vi "Export Custom Device Configuration.vi"(8 "error in (no error)":errorcluster, 11 "Node Ptr":u64 format="%.0x") -> (0 "error out":errorcluster)   [LabVIEW 2015, in "Import Export Sample Custom Device System Explorer.lvlib"]
uses:
  Import Export Sample Custom Device System Explorer.lvlib
  <vilib>/NI/NIVS System Definition Utilities/System Definition Utilities.lvlib
panel:
  in  "Tag":string
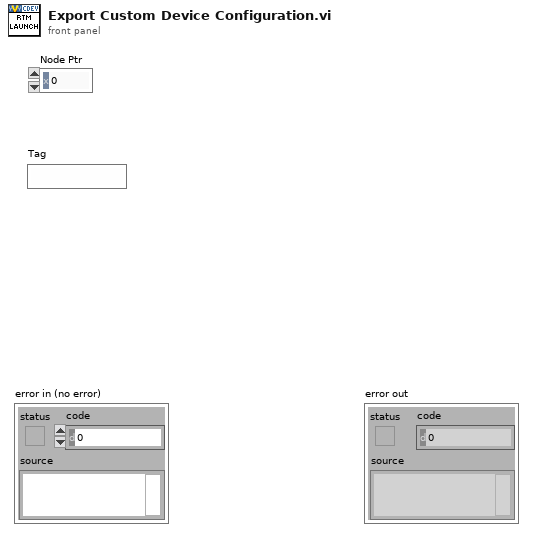
[diagram p1: front panel]
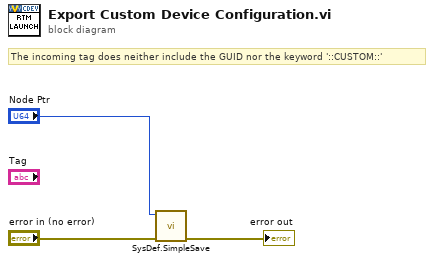
[diagram p0: block diagram]
diagram:
  # "The incoming tag does neither include the GUID nor the keyword '::CUSTOM::'"
  n1 = call <vilib>:"SysDef.SimpleSave.vi"("error in (no error)"="error in (no error)", "ID"="Node Ptr") -> ("error out"=→"error out":errorcluster)  [unwired: 8 in, 1 out]
